vi "EOL CAN_Target Motion.vi"(7 "Rx Arbitration Id":u32=402522244 format="%.0x", 8 "Error in":errorcluster, 9 "All Motions":T1, 10 "Read Session in":refnum<k21>, 11 "Write Session in":refnum<k21>) -> (0 "Error out":errorcluster, 2 "TxRx Data":string[][](array[string]), 3 "Response Good?":bool)   [LabVIEW 2014]
uses:
  typedefs/All Motions.ctl
  <vilib>/xnet/xnet.llb/XNET Frame CAN.ctl
  <vilib>/xnet/xnet.llb/XNET Frame Type CAN.ctl
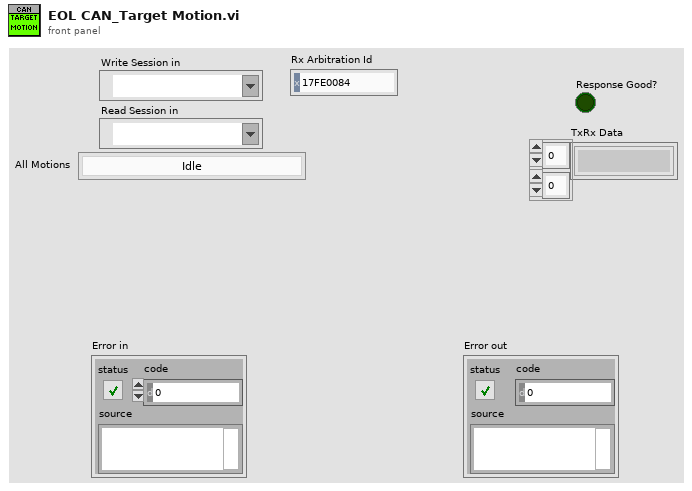
[diagram p1: front panel]
types:
  T1 = typedef "All Motions.ctl" = enum16{"Idle", "Glass Teach", "Glass Slide Open", "Glass Slide Open 2", "Glass Slide Close", "Glass Slide Close 2", "Glass Vent Open", "Glass Vent Close", "Sunshade Teach", "Sunshade Teach 2", "Sunshade Open", "Sunshade Open 2", "Sunshade Close", "Sunshade Close 2", "Glass Slide Open Sunshade Open", "Glass Slide Open 2 Sunshade Open", "Glass Slide Open Sunshade Close", "Glass Slide Open 2 Sunshade Close", "Glass Slide Close Sunshade Open", "Glass Slide Close 2 Sunshade Open", "Glass Slide Close Sunshade Close", "Glass Slide Close 2 Sunshade Close", "Glass Vent Open Sunshade Open", "Glass Vent Open Sunshade Close", "Glass Vent Close Sunshade Open", "Glass Vent Close Sunshade Close", "Express Glass Slide Open", "Express Glass Slide Open 2", "Express Glass Slide Close", "Express Glass Slide Close 2", "Express Glass Vent Open", "Express Glass Vent Close", "Express Sunshade Open", "Express Sunshade Close", "Express Sunshade Open 2", "Express Sunshade Close 2", "Express Glass Slide Open Sunshade Open", "Express Glass Slide Open 2 Sunshade Open", "Express Glass Slide Open Sunshade Close", "Express Glass Slide Open 2 Sunshade Close", "Express Glass Slide Close Sunshade Open", "Express Glass Slide Close 2 Sunshade Open", "Express Glass Slide Close Sunshade Close", "Express Glass Slide Close 2 Sunshade Close", "Express Glass Vent Open Sunshade Open", "Express Glass Vent Open Sunshade Close", "Express Glass Vent Close Sunshade Open", "Express Glass Vent Close Sunshade Close", "Goto Position Glass", "Goto Position Sunshade"}
  T2 = typedef "XNET Frame CAN.ctl" = cluster{"timestamp":timestamp, "payload":u8[], "identifier":u32, "type":T3, "extended?":bool, "echo?":bool}
  T3 = typedef "XNET Frame Type CAN.ctl" = u8
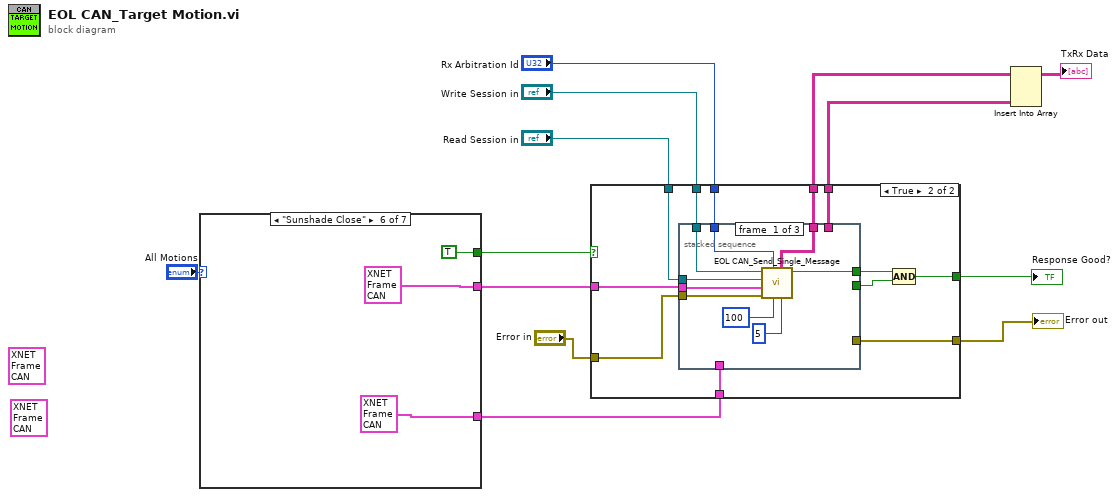
[diagram p0: block diagram]
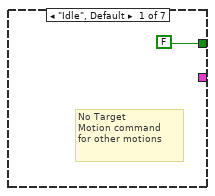
[diagram p2: hidden frame]
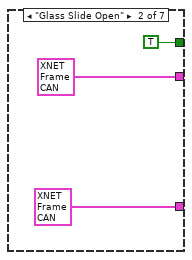
[diagram p3: hidden frame]
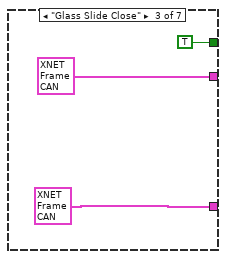
[diagram p4: hidden frame]
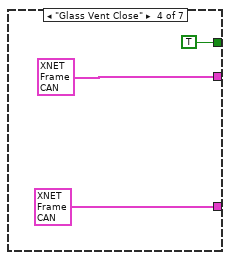
[diagram p5: hidden frame]
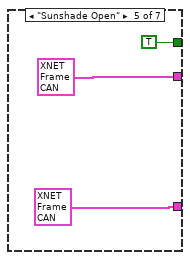
[diagram p6: hidden frame]
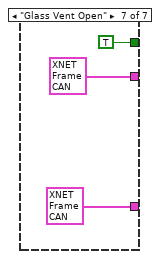
[diagram p7: hidden frame]
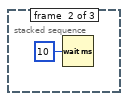
[diagram p9: hidden frame]
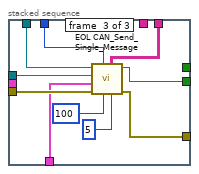
[diagram p10: hidden frame]
diagram:
  (unwired) T2 {"timestamp"=timestamp(0 s since 1904-01-01), "payload"=[6, 49, 1, 16, 0, 0, 176, 85], "identifier"=402391172, "type"=8, "extended?"=TRUE, "echo?"=FALSE} ("Tx CAN frame")
  (unwired) T2 {"timestamp"=timestamp(0 s since 1904-01-01), "payload"=[7, 35, 20, 64, 0, 68, 250, 2], "identifier"=402391172, "type"=8, "extended?"=TRUE, "echo?"=FALSE} ("Tx CAN frame")
  n1 = case shown="\"Sunshade Close\"" "All Motions" {
    tunnel: [_ T2 {"timestamp"=timestamp(0 s since 1904-01-01), "payload"=[2, 16, 79, 85, 85, 85, 85, 85], "identifier"=402391172, "type"=8, "extended?"=TRUE, "echo?"=FALSE} ("Tx CAN frame") T2 {"timestamp"=timestamp(0 s since 1904-01-01), "payload"=[2, 16, 79, 85, 85, 85, 85, 85], "identifier"=402391172, "type"=8, "extended?"=TRUE, "echo?"=FALSE} ("Tx CAN frame") T2 {"timestamp"=timestamp(0 s since 1904-01-01), "payload"=[2, 16, 79, 85, 85, 85, 85, 85], "identifier"=402391172, "type"=8, "extended?"=TRUE, "echo?"=FALSE} ("Tx CAN frame") T2 {"timestamp"=timestamp(0 s since 1904-01-01), "payload"=[2, 16, 79, 85, 85, 85, 85, 85], "identifier"=402391172, "type"=8, "extended?"=TRUE, "echo?"=FALSE} ("Tx CAN frame") T2 {"timestamp"=timestamp(0 s since 1904-01-01), "payload"=[2, 16, 79, 85, 85, 85, 85, 85], "identifier"=402391172, "type"=8, "extended?"=TRUE, "echo?"=FALSE} ("Tx CAN frame") T2 {"timestamp"=timestamp(0 s since 1904-01-01), "payload"=[2, 16, 79, 85, 85, 85, 85, 85], "identifier"=402391172, "type"=8, "extended?"=TRUE, "echo?"=FALSE} ("Tx CAN frame")] -> w8
    tunnel: [_ T2 {"timestamp"=timestamp(0 s since 1904-01-01), "payload"=[6, 47, 128, 90, 3, 255, 16, 85], "identifier"=402391172, "type"=8, "extended?"=TRUE, "echo?"=FALSE} ("Tx CAN frame") T2 {"timestamp"=timestamp(0 s since 1904-01-01), "payload"=[6, 47, 128, 90, 3, 255, 48, 85], "identifier"=402391172, "type"=8, "extended?"=TRUE, "echo?"=FALSE} ("Tx CAN frame") T2 {"timestamp"=timestamp(0 s since 1904-01-01), "payload"=[6, 47, 128, 90, 3, 255, 48, 85], "identifier"=402391172, "type"=8, "extended?"=TRUE, "echo?"=FALSE} ("Tx CAN frame") T2 {"timestamp"=timestamp(0 s since 1904-01-01), "payload"=[6, 47, 128, 91, 3, 255, 16, 85], "identifier"=402391172, "type"=8, "extended?"=TRUE, "echo?"=FALSE} ("Tx CAN frame") T2 {"timestamp"=timestamp(0 s since 1904-01-01), "payload"=[6, 47, 128, 91, 3, 255, 32, 85], "identifier"=402391172, "type"=8, "extended?"=TRUE, "echo?"=FALSE} ("Tx CAN frame") T2 {"timestamp"=timestamp(0 s since 1904-01-01), "payload"=[6, 47, 128, 90, 3, 255, 32, 85], "identifier"=402391172, "type"=8, "extended?"=TRUE, "echo?"=FALSE} ("Tx CAN frame")] -> w2
    tunnel: [FALSE TRUE TRUE TRUE TRUE TRUE TRUE] -> w1
    frame "Idle", Default {
      # "No Target\nMotion command\nfor other motions"
    }
    frame "Glass Slide Open" {
    }
    frame "Glass Slide Close" {
    }
    frame "Glass Vent Close" {
    }
    frame "Sunshade Open" {
    }
    frame "Sunshade Close" {
    }
    frame "Glass Vent Open" {
    }
  }
  n2 = case shown="True" w1 {
    selector: w1 -> [w34 _]
    tunnel: "Error in" -> [w33 w46]
    tunnel: [w33 w45] -> w12
    tunnel: "Rx Arbitration Id" -> [_ w44]
    tunnel: "Write Session in" -> [_ w43]
    tunnel: "Read Session in" -> [_ w42]
    tunnel: w8 -> [_ w41]
    tunnel: [_ w40] -> w5
    tunnel: [_ w39] -> w4
    tunnel: [w34 w38] -> w3
    tunnel: w2 -> [_ w35]
    frame False {
    }
    frame True {
      n3 = stacked-sequence {
        tunnel: w46 -> [w55 _ w66]
        tunnel: [_ _ w60] -> w45
        tunnel: [w54 _ _] -> w40
        tunnel: w44 -> [w53 _ w65]
        tunnel: w43 -> [w52 _ w64]
        tunnel: w42 -> [w51 _ w63]
        tunnel: [w50 _ _] -> w37
        tunnel: w41 -> [w47 _ _]
        tunnel: [_ _ w59] -> w39
        tunnel: [_ _ w58] -> w36
        tunnel: w35 -> [_ _ w57]
        frame #0 {
          n4 = call "EOL CAN_Send_Single_Message.vi"("Retries"=5, "Msg Wait Time"=u32 100, "Rx Arbitration Id"=w53, "Error in"=w55, "Tx CAN frame"=w47, "Read Session in"=w51, "Write Session in"=w52) -> ("Response Good?"=w50:bool, "TxRx Data"=w54:string[][])  [unwired: 3 out]
        }
        frame #1 {
          n5 = Wait (ms)(milliseconds to wait=u32 10) -> ()  [unwired: 1 out]
        }
        frame #2 {
          n6 = call "EOL CAN_Send_Single_Message.vi"("Retries"=5, "Msg Wait Time"=u32 100, "Rx Arbitration Id"=w65, "Error in"=w66, "Tx CAN frame"=w57, "Read Session in"=w63, "Write Session in"=w64) -> ("Error out"=w60:errorcluster, "Response Good?"=w58:bool, "TxRx Data"=w59:string[][])  [unwired: 2 out]
        }
      }
      n7 = Compound Arithmetic op=AND(w37, w36) -> (w38:bool)
    }
  }
  "Error out" <- w12
  "Response Good?" <- w3
  n8 = Insert Into Array(array=w5, new element=w4) -> (→"TxRx Data":string[][])  [unwired: 2 in]
